vi "Delete DVR_Queue.vi"(0 "Queue DVR in":refnum<data-value>, 11 "error in (no error)":errorcluster) -> (15 "error out":errorcluster)   [LabVIEW 2020, in "Data Communication Transmitter.lvlib" / "Queue.lvclass"]
uses:
  Classes/Children/Intra-Application/Children/With Data/Children/Queues/Queue.lvclass
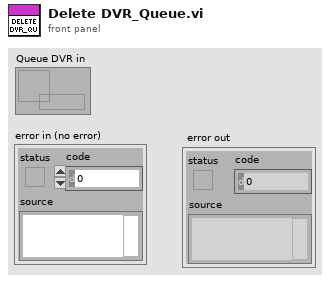
[diagram p1: front panel]
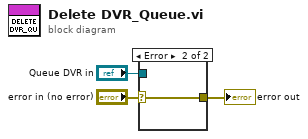
[diagram p0: block diagram]
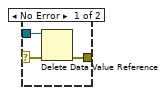
[diagram p2: hidden frame]
diagram:
  n1 = case shown="Error" "error in (no error)" {
    selector: "error in (no error)" -> [w6 w7]
    tunnel: [w5 w7] -> w2
    tunnel: "Queue DVR in" -> [w4 _]
    frame No Error {
      n2 = Delete Data Value Reference(data value reference=w4, error in=w6) -> (error out=w5:errorcluster)  [unwired: 1 out]
    }
    frame Error {
    }
  }
  "error out" <- w2
